vi "RDV-singleGraph-SelectData.vi"(8 "error in (no error)":errorcluster, 11 "RDV-Reflection_Data_viewer in":refnum<class "RDV-Reflection_Data_viewer.lvclass">) -> (0 "error out":errorcluster, 3 "RDV-Reflection_Data_viewer out":refnum<class "RDV-Reflection_Data_viewer.lvclass">)   [LabVIEW 2020, in "RDV-Reflection_Data_viewer.lvclass"]
uses:
  RDV-Reflection_Data_viewer.lvclass
  RDV-Reflection_Data_viewer.lvclass/RDV-Reflection_Data_viewer.ctl
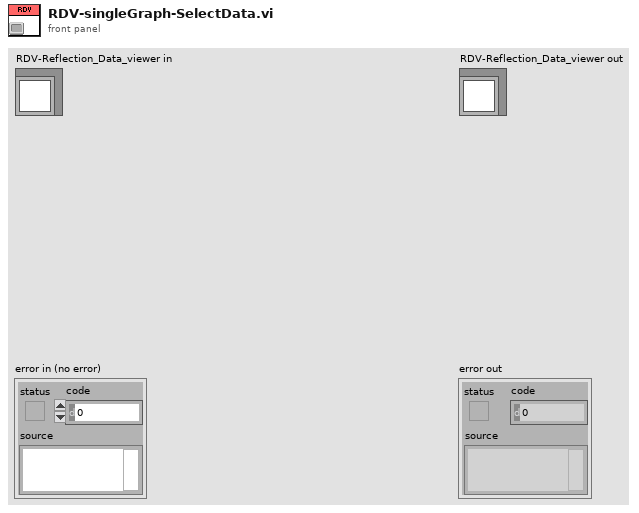
[diagram p1: front panel]
types:
  T1 = cluster{"Frequency":dbl[], "Reflection'":dbl[]}[]
  T2 = cluster{"Frequency":dbl[], "Reflection'":dbl[]}[][]
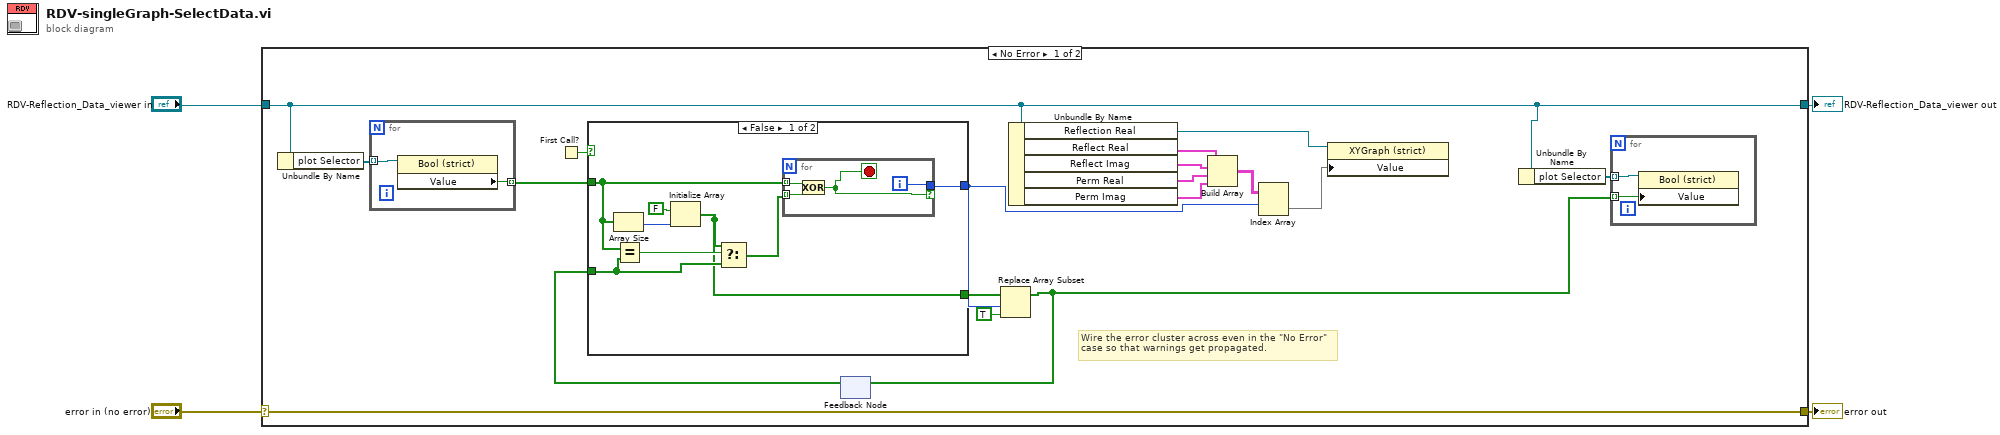
[diagram p0: block diagram]
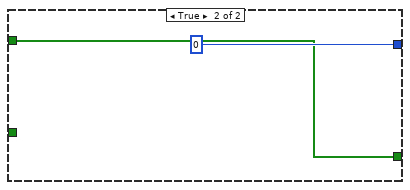
[diagram p2: hidden frame]
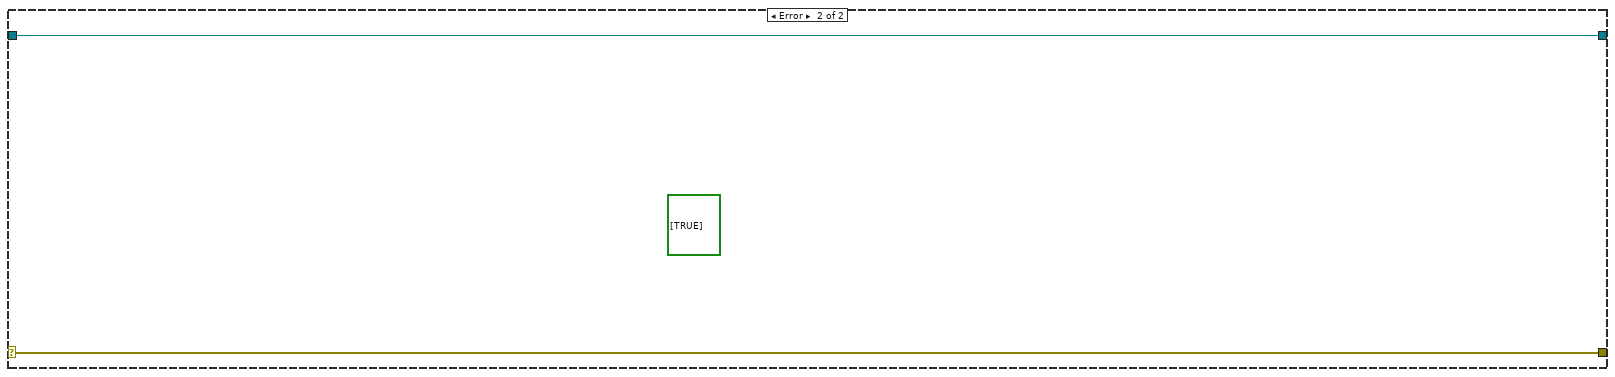
[diagram p3: hidden frame]
diagram:
  n1 = case shown="No Error" "error in (no error)" {
    selector: "error in (no error)" -> [w22 w42]
    tunnel: [w22 w42] -> w3
    tunnel: [w6 w41] -> w1
    tunnel: "RDV-Reflection_Data_viewer in" -> [w6 w41]
    frame No Error {
      # "Wire the error cluster across even in the \"No Error\"\ncase so that warnings get propagated."
      n2 = Unbundle By Name(w6) -> ("plot Selector"=w9:refnum<vi>[])
      n3 = for {
        tunnel: w9 -> [w26] mode=indexing
        tunnel: [w25] -> w8 mode=indexing
        n4 = property on="Property Node" class="Bool (strict)"(reference=w26) -> ("Value"=w25:bool)  [unwired: 1 in, 2 out]
      }
      n5 = First Call?() -> (First Call?: T/F=w11:bool)
      n6 = feedback #1() -> (w10:bool[])  [unwired: 1 in]
      n7 = case shown="False" w11 {
        tunnel: [w28 w39] -> w14
        tunnel: [w32 0] -> w13
        tunnel: w8 -> [w31 w39]
        tunnel: w10 -> [w29 _]
        frame False {
          n8 = Array Size(array=w31) -> (size(s)=w34:i32)
          n9 = Equal?(x=w31, y=w29) -> (x = y?=w30:bool)
          n10 = Initialize Array(FALSE, w34) -> (w28:bool[])
          n11 = Select(t=w28, s=w30, f=w29) -> (s? t:f=w27:bool[])
          n12 = for {
            tunnel: w31 -> [w37] mode=indexing
            tunnel: [w38] -> w32 if=w35
            tunnel: w27 -> [w36] mode=indexing
            i -> [w38]
            stop <- w35 stop-if-true
            n13 = Exclusive Or(1:w36, 2:w37) -> (0:w35:bool)
          }
        }
        frame True {
        }
      }
      n14 = Replace Array Subset(array=w14, new element=TRUE ("new element/subarray"), index=w13) -> (w5:bool[])
      n15 = feedback-in #1(w5) -> ()
      n16 = Unbundle By Name(w6) -> ("Reflection Real"=w17:refnum<vi>, "Reflect Real"=w21:T1, "Reflect Imag"=w20:T1, "Perm Real"=w19:T1, "Perm Imag"=w18:T1)
      n17 = Build Array(w21, w20, w19, w18) -> (w16:T2)
      n18 = Index Array(array=w16, index (row)=w13) -> (element=w15:T1)  [unwired: 1 in]
      n19 = property on="Property Node" class="XYGraph (strict)"(reference=w17, "Value"=w15) -> ()  [unwired: 1 in, 2 out]
      n20 = Unbundle By Name(w6) -> ("plot Selector"=w7:refnum<vi>[])
      n21 = for {
        tunnel: w7 -> [w24] mode=indexing
        tunnel: w5 -> [w23] mode=indexing
        n22 = property on="Property Node" class="Bool (strict)"(reference=w24, "Value"=w23) -> ()  [unwired: 1 in, 2 out]
      }
    }
    frame Error {
      (unwired) bool[] [TRUE]
    }
  }
  "error out" <- w3
  "RDV-Reflection_Data_viewer out" <- w1
